vi "Initialize.vi"(8 "error in":errorcluster, 11 "TSI 3071 in":refnum<class "TSI 3071.lvclass">) -> (0 "error out":errorcluster, 3 "TSI 3071 out":refnum<class "TSI 3071.lvclass">)   [LabVIEW 2015, in "TSI 3071.lvclass"]
uses:
  TSI 3071.lvclass
  DMA.lvclass/DMA.ctl
  Accessors/Write ri.vi
  Accessors/Write ro.vi
  Accessors/Write Leff.vi
  DMA.lvclass
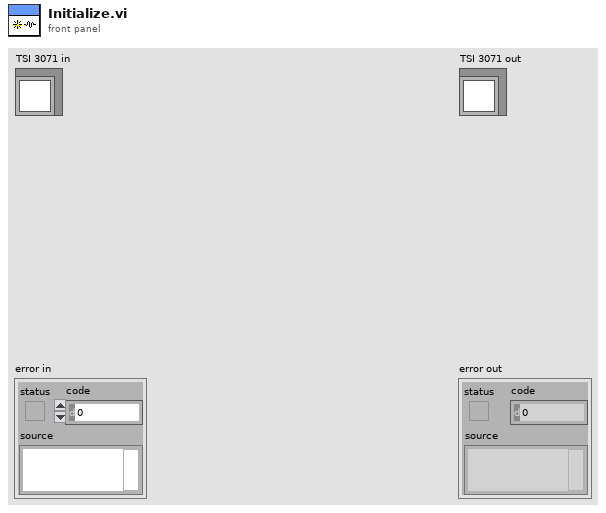
[diagram p1: front panel]
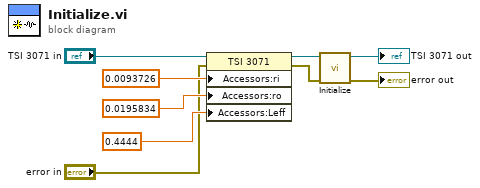
[diagram p0: block diagram]
diagram:
  n1 = property class="TSI 3071"(reference="TSI 3071 in", error in="error in", "Accessors:ri"=0.0093726 ("ri"), "Accessors:ro"=0.0195834 ("ro"), "Accessors:Leff"=0.4444 ("Leff")) -> (reference out=w9:refnum<class "TSI 3071.lvclass">, error out=w5:errorcluster)
  n2 = call-parent "Initialize.vi"("error in"=w5, "DMA in"=w9) -> ("error out"=→"error out":errorcluster, "DMA out"=→"TSI 3071 out":refnum<class "TSI 3071.lvclass">)  [unwired: 8 in]
